vi "Root Info.vi"(11 "Value Tree in":refnum<class "Value Tree.lvclass">) -> (1 "Type":T1, 2 "Value":string, 3 "Value Tree out":refnum<class "Value Tree.lvclass">, 5 "Children":string[](array[string]), 7 "Size":i32)   [LabVIEW 2020, in "HTTP Server.lvlib" / "Value Tree.lvclass"]
uses:
  Value Tree.lvclass
  Value Tree.lvclass/Value Tree.ctl
  Local Type.ctl
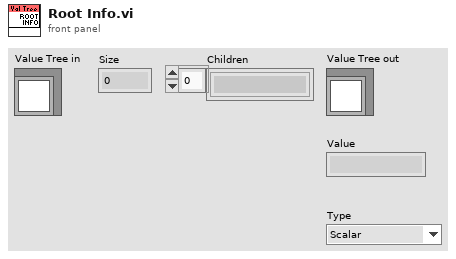
[diagram p1: front panel]
types:
  T1 = typedef "HTTP Server.lvlib/Value Tree.lvclass/Local Type.ctl" = enum16{"Scalar", "Object", "Array"}
  T2 = typedef "HTTP Server.lvlib/Value Tree.lvclass/Local Info.ctl" = cluster{"Type":T1, "Value":string, "Children":string[], "Size":i32}
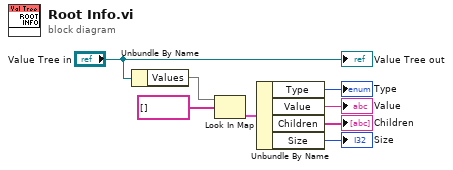
[diagram p0: block diagram]
diagram:
  n1 = Unbundle By Name("Value Tree in") -> ("Values"=w7:map{string[], T2})
  n2 = Look In Map(map=w7, key=string[] []) -> (value=w5:T2)  [unwired: 1 in, 1 out]
  n3 = Unbundle By Name(w5) -> ("Type"=→"Type":T1, "Value"=→"Value":string, "Children"=→"Children":string[], "Size"=→"Size":i32)
  "Value Tree out" <- "Value Tree in"
